vi "Auto Ground Manipulator Command.vi"(8 "Command Info In":T1, 11 "intake modes":T4) -> (0 "Command Info Out":T1)   [LabVIEW 2020]
uses:
  intake sub/Implementation/Typedef/intake typedef.ctl
  <vilib>/Rock Robotics/WPI/Framework/Command Status Info.ctl
  <vilib>/Rock Robotics/WPI/Framework/Completion Status.ctl
  <vilib>/Rock Robotics/WPI/Framework/Completion Notifier.ctl
  Implementation/Typedefs/game object.ctl
  Implementation/Typedefs/Teleop Manipulator Commands.ctl
  Framework/Robot Global Data.vi
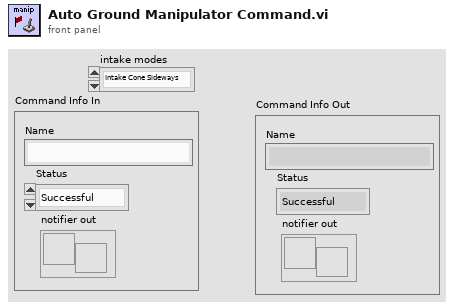
[diagram p1: front panel]
types:
  T1 = typedef "Command Status Info.ctl" = cluster{"Name":string, "Status":T2, "notifier out":T3}
  T2 = typedef "Completion Status.ctl" = enum16{"Successful", "Aborted", "Incomplete"}
  T3 = typedef "Completion Notifier.ctl" = refnum<notifier>
  T4 = typedef "intake typedef.ctl" = enum16{"Intake Cone Sideways", "Intake Cone Upright", "Intake Cube", "Outtake/Score"}
  T5 = typedef "Teleop Manipulator Commands.ctl" = enum16{"idle", "intake cone sideways", "intake cone upright", "intake cube", "score low cone", "score low cube", "score mid cone", "score mid cube", "score high cone", "score high cube"}
  T6 = typedef "game object.ctl" = enum16{"Nothing", "Cone", "Cube"}
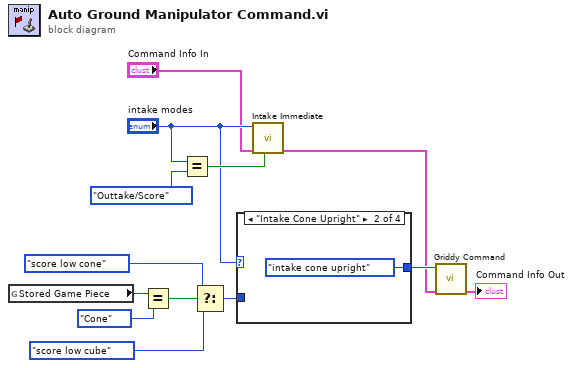
[diagram p0: block diagram]
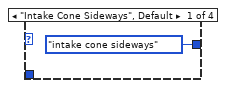
[diagram p2: hidden frame]
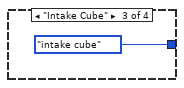
[diagram p3: hidden frame]
diagram:
  n1 = global read "Robot Global Data.vi" "Stored Game Piece"() -> (w9:T6)
  n2 = Equal?(x=w9, y=game_object."Cone") -> (x = y?=w7:bool)
  n3 = Equal?(x="intake modes", y=intake_typedef."Outtake/Score") -> (x = y?=w12:bool)
  n4 = Select(t=Teleop_Manipulator_Commands."score low cone" ("Griddy Command"), s=w7, f=Teleop_Manipulator_Commands."score low cube" ("Griddy Command")) -> (s? t:f=w4:T5)
  n5 = case shown="\"Intake Cone Upright\"" "intake modes" {
    tunnel: [Teleop_Manipulator_Commands."intake cone sideways" ("Griddy Command") Teleop_Manipulator_Commands."intake cone upright" ("Griddy Command") Teleop_Manipulator_Commands."intake cube" ("Griddy Command") w17] -> w10
    tunnel: w4 -> [_ _ _ w17]
    frame "Intake Cone Sideways", Default {
    }
    frame "Intake Cone Upright" {
    }
    frame "Intake Cube" {
    }
    frame "Outtake/Score" {
    }
  }
  n6 = call "Intake Immediate.vi"("Wait for Manipulator"=w12, "Command Info In"="Command Info In", "intake modes"="intake modes") -> ("Command Info Out"=w3:T1)  [unwired: 8 in]
  n7 = call "Griddy Command.vi"("Command Info In"=w3, "Griddy Command"=w10) -> ("Command Info Out"=→"Command Info Out":T1)  [unwired: 9 in]
